vi "create.vi"(8 "error in":errorcluster, 10 "client":string="NotAuniqueID", 11 "URI":string="tcp://iot.eclipse.org:1883") -> (0 "error out":errorcluster, 3 "MQTT client out":refnum<class "MQTT client.lvclass">)   [LabVIEW 2014, in "MQTT client.lvclass"]
uses:
  MQTT client.lvclass
  status event.ctl
  subscribed message.ctl
  message acknowledgement.ctl
  MQTT client.lvclass/MQTT client.ctl
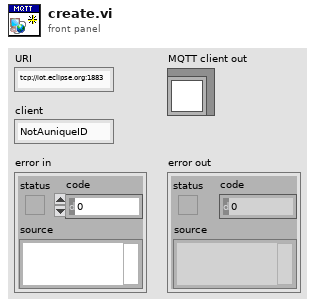
[diagram p1: front panel]
types:
  T1 = typedef "MQTT client.lvclass/message acknowledgement.ctl" = i32
  T2 = typedef "MQTT client.lvclass/status event.ctl" = cluster{"code":i32, "message":string}
  T3 = typedef "MQTT client.lvclass/subscribed message.ctl" = cluster{"ID":i32, "topic":string, "data":string}
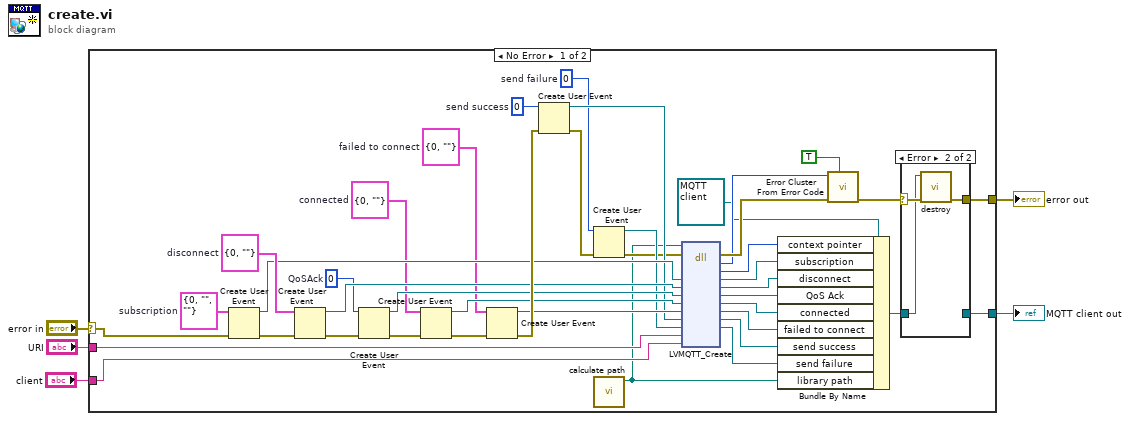
[diagram p0: block diagram]
diagram:
  n1 = case shown="No Error" "error in" {
    selector: "error in" -> [w17 w52]
    tunnel: [w15 w52] -> w4
    tunnel: [w14 _] -> w1
    tunnel: "URI" -> [w9 _]
    tunnel: "client" -> [w8 _]
    frame No Error {
      w22 = T1 0  # send failure
      w21 = T1 0  # send success
      w23 = T2 {"code"=0, "message"=""}  # failed to connect
      w29 = T2 {"code"=0, "message"=""}  # connected
      w32 = T1 0  # QoSAck
      w36 = T3 {"ID"=0, "topic"="", "data"=""}  # subscription
      w37 = T2 {"code"=0, "message"=""}  # disconnect
      n2 = Create User Event(user event datatype=w36, error in=w17) -> (user event=w35:refnum<user-event>, error out=w44:errorcluster)
      n3 = Create User Event(user event datatype=w37, error in=w44) -> (user event=w38:refnum<user-event>, error out=w43:errorcluster)
      n4 = Create User Event(user event datatype=w32, error in=w43) -> (user event=w31:refnum<user-event>, error out=w42:errorcluster)
      n5 = Create User Event(user event datatype=w29, error in=w42) -> (user event=w28:refnum<user-event>, error out=w41:errorcluster)
      n6 = Create User Event(user event datatype=w23, error in=w41) -> (user event=w26:refnum<user-event>, error out=w40:errorcluster)
      n7 = Create User Event(user event datatype=w21, error in=w40) -> (user event=w25:refnum<user-event>, error out=w39:errorcluster)
      n8 = Create User Event(user event datatype=w22, error in=w39) -> (user event=w24:refnum<user-event>, error out=w7:errorcluster)
      n9 = call "calculate path.vi"() -> ("Path"=w6:path)  [unwired: 11 in]
      n10 = dll-call lib="paho-mqtt3a.dll" fn="LVMQTT_Create"(path in=w6, error in=w7, "subMsg"=w35, "disconnect"=w38, "QoSAck"=w31, "connSuccess"=w28, "connFail"=w26, "sendS"=w25, "sendF"=w24, "URI"=w9, "client"=w8) -> (error out=w46:errorcluster, "return type"=w45:i32, "lvctx"=w11:u64, "subMsg"=w33:refnum<user-event>, "disconnect"=w34:refnum<user-event>, "QoSAck"=w30:refnum<user-event>, "connSuccess"=w27:refnum<user-event>, "connFail"=w18:refnum<user-event>, "sendS"=w19:refnum<user-event>, "sendF"=w20:refnum<user-event>)  [unwired: 4 in, 1 out]
      n11 = Bundle By Name(cluster=refnum<class "MQTT client.lvclass"> refnum ("MQTT client in"), "context pointer"=w11, "subscription"=w33, "disconnect"=w34, "QoS Ack"=w30, "connected"=w27, "failed to connect"=w18, "send success"=w19, "send failure"=w20, "library path"=w6) -> (w12:refnum<class "MQTT client.lvclass">)
      n12 = call <vilib>:"Error Cluster From Error Code.vi"("show call chain? (False)"=TRUE, "error in (no error)"=w46, "error code (0)"=w45) -> ("error out"=w16:errorcluster)  [unwired: 6 in]
      n13 = case shown="Error" w16 {
        selector: w16 -> [w48 w51]
        tunnel: [w48 w50] -> w15
        tunnel: w12 -> [w47 w49]
        tunnel: [w47 _] -> w14
        frame No Error {
        }
        frame Error {
          n14 = call "destroy.vi"("error in"=w51, "MQTT client in"=w49) -> ("error out"=w50:errorcluster)  [unwired: 9 in]
        }
      }
    }
    frame Error {
    }
  }
  "error out" <- w4
  "MQTT client out" <- w1
